vi "Set.vi"(0 "S_Call_Function":string="outputVoltage", 1 "S_Channel":string="0", 2 "IP":string="192.168.0.250", 3 "Data_type":string="F", 4 "Value":string="100") -> (5 "S_Return":string)   [LabVIEW 2018]
panel:
  out "Full Command":string
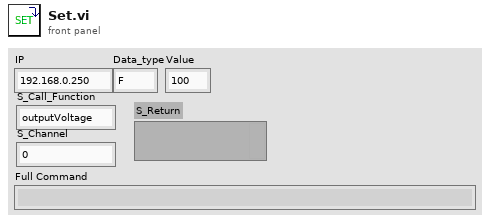
[diagram p1: front panel]
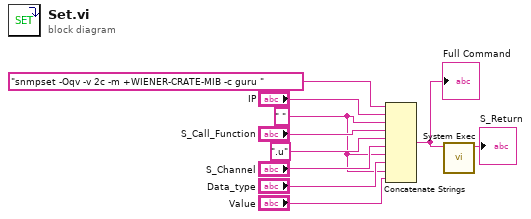
[diagram p0: block diagram]
diagram:
  w2 = " "
  n1 = Concatenate Strings("snmpset -Oqv -v 2c -m +WIENER-CRATE-MIB -c guru ", "IP", w2, "S_Call_Function", ".u", "S_Channel", w2, "Data_type", w2, "Value") -> (w5:string)
  "Full Command" <- w5
  n2 = call <vilib>:"System Exec.vi"("command line"=w5) -> ("standard output"=→"S_Return":string)  [unwired: 7 in, 3 out]
